vi "startUp.vi"(8 "error in (no error)":errorcluster, 11 "StaticOutputEditor.lvclass":refnum<class "StaticOutputEditor.lvclass">) -> (0 "error out":errorcluster, 3 "StaticOutputEditor.lvclass 2":refnum<class "StaticOutputEditor.lvclass">)   [LabVIEW 2011, in "Views.lvlib" / "ScriptEditor.lvlib" / "StaticOutputEditor.lvclass"]
uses:
  StaticOutputEditor.lvclass
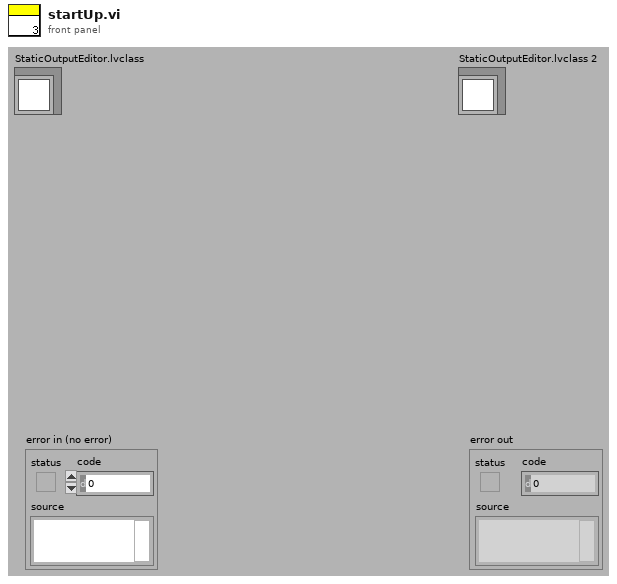
[diagram p1: front panel]
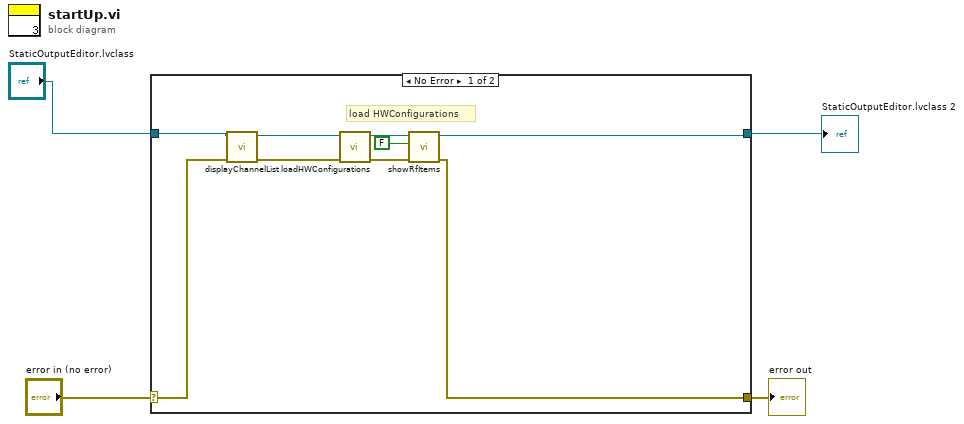
[diagram p0: block diagram]
diagram:
  n1 = case shown="No Error" "error in (no error)" {
    selector: "error in (no error)" -> [w12 w15]
    tunnel: [w6 w15] -> w3
    tunnel: [w7 w14] -> w1
    tunnel: "StaticOutputEditor.lvclass" -> [w13 w14]
    frame No Error {
      # "load HWConfigurations"
      n2 = call "displayChannelList.vi"("error in (no error)"=w12, "StaticOutputEditor in"=w13) -> ("error out"=w10:errorcluster, "StaticOutputEditor out"=w11:refnum<class "StaticOutputEditor.lvclass">)  [unwired: 8 in]
      n3 = call "loadHWConfigurations.vi"("error in (no error)"=w10, "StaticOutputEditor in"=w11) -> ("error out"=w8:errorcluster, "StaticOutputEditor out"=w9:refnum<class "StaticOutputEditor.lvclass">)  [unwired: 8 in]
      n4 = call "showRfItems.vi"("error in (no error)"=w8, "show/hide"=FALSE, "StaticOutputEditor in"=w9) -> ("error out"=w6:errorcluster, "StaticOutputEditor out"=w7:refnum<class "StaticOutputEditor.lvclass">)  [unwired: 7 in]
    }
    frame Error {
    }
  }
  "error out" <- w3
  "StaticOutputEditor.lvclass 2" <- w1
